vi "read_usalex_photon_hdf5.vi"() -> ()   [LabVIEW 2010]
uses:
  <vilib>/addons/h5labview2/file/H5F.lvlib
  <vilib>/addons/h5labview2/file/H5Fmode.ctl
  <vilib>/addons/h5labview2/group/H5G.lvlib
  <vilib>/addons/h5labview2/dataset/H5Dread.llb/H5Dread.xnode
  <vilib>/addons/h5labview2/base/H5Equery.vi
  <vilib>/addons/h5labview2/base/lib_path.vi
  <vilib>/Analysis/NI_AALBase.lvlib
  <vilib>/Analysis/1siggen.llb/Ramp Pattern by Delta.vi
  <vilib>/addons/h5labview2/base/hid_t.ctl
panel:
  out "measurement_type":string
  out "error out":errorcluster
  out "ALEX Histograms":cluster{"Ramp Pattern":dbl[], u32[]}[](graph)
  out "acceptor_period":u32[](array[numeric])
  out "donor_period":u32[](array[numeric])
  out "alex_offset":u32
  out "alex_period":u32
  out "spectral_ch2":u32[](array[numeric])
  out "spectral_ch1":u32[](array[numeric])
  out "detectors":u32[](array[numeric])
  out "timestamps_unit":dbl
  out "timestamps":i64[](array[numeric])
  in  "Path":path
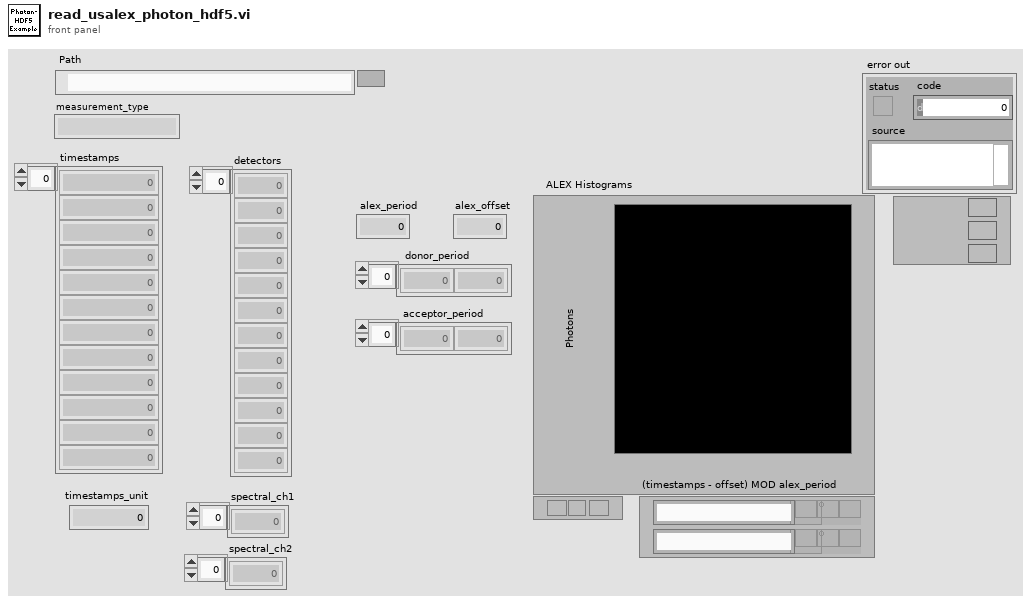
[diagram p1: front panel]
types:
  T1 = typedef "H5F.lvlib/H5Fmode.ctl" = enum16{"read-only", "read-write", "overwrite", "create new", "open or create"}
  T2 = typedef "hid_t.ctl" = i32
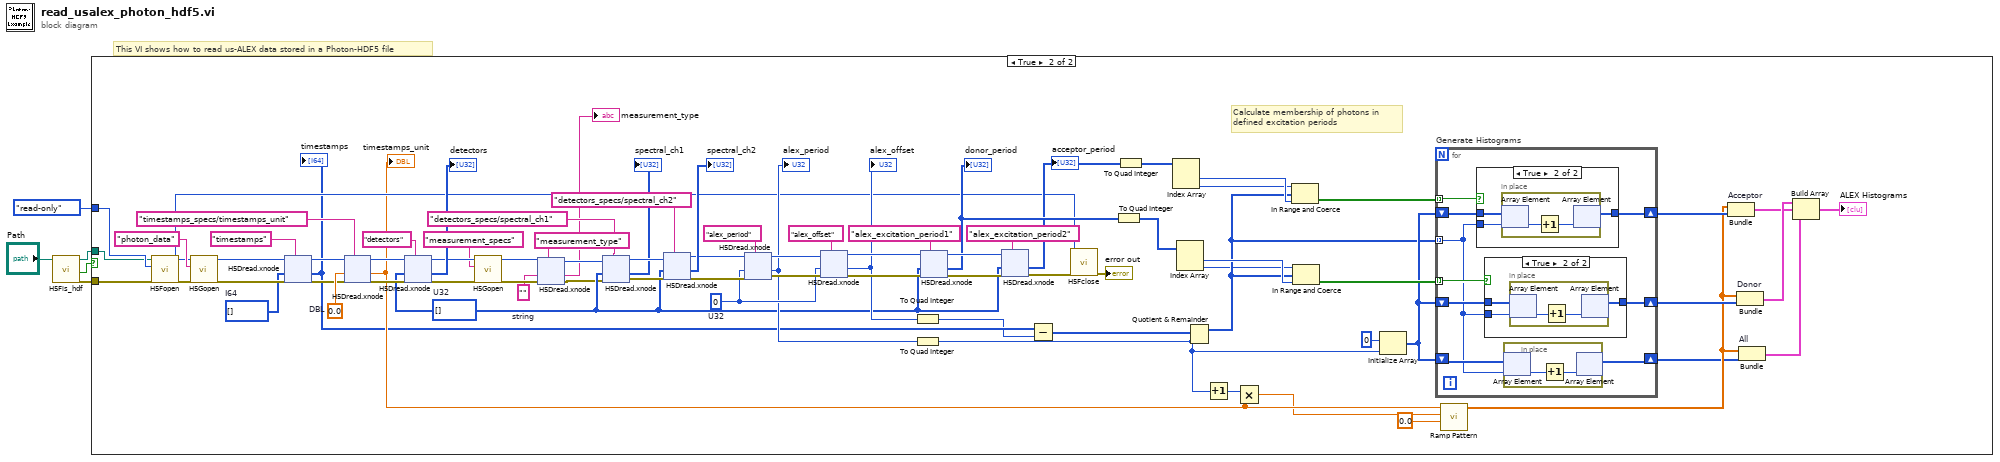
[diagram p0: block diagram]
diagram:
  # "This VI shows how to read us-ALEX data stored in a Photon-HDF5 file"
  n1 = call <vilib>:"H5Fis_hdf.vi"("path in"="Path") -> ("error out"=w1:errorcluster, "valid?"=w2:bool, "path out"=w3:path)  [unwired: 7 in, 1 out]
  n2 = case shown="True" w2 {
    tunnel: H5Fmode."read-only" ("mode (read-only)") -> [_ w86]
    tunnel: w3 -> [_ w85]
    tunnel: w1 -> [_ w84]
    frame False {
    }
    frame True {
      w7 = ""  # string
      w54 = u32 0  # U32
      w37 = u32[] []  # U32
      w77 = 0.0  # DBL
      w78 = i64[] []  # I64
      # "Calculate membership of photons in\ndefined excitation periods"
      n3 = call <vilib>:"H5Fopen.vi"("error in (no error)"=w84, "mode (read-only)"=w86, "path"=w85) -> ("error out"=w83:errorcluster, "ref out"=w32:T2)  [unwired: 7 in]
      n4 = call <vilib>:"H5Gopen.vi"("error in (no error)"=w83, "name"="photon_data", "ref in"=w32) -> ("error out"=w79:errorcluster, "group out"=w81:T2)  [unwired: 7 in]
      n5 = xnode "H5Dread.xnode"("dataset name (this)"="timestamps", "error in (no error)"=w79, "default"=w78, "ref in"=w81) -> ("error out"=w75:errorcluster, "data"=w17:i64[], "ref out"=w76:i32)  [unwired: 2 in, 1 out]
      "timestamps" <- w17
      n6 = xnode "H5Dread.xnode"("dataset name (this)"="timestamps_specs/timestamps_unit" ("object name"), "error in (no error)"=w75, "default"=w77, "ref in"=w76) -> ("error out"=w70:errorcluster, "data"=w29:dbl, "ref out"=w71:i32)  [unwired: 2 in, 1 out]
      "timestamps_unit" <- w29
      n7 = xnode "H5Dread.xnode"("dataset name (this)"="detectors", "error in (no error)"=w70, "default"=w37, "ref in"=w71) -> ("error out"=w67:errorcluster, "data"=→"detectors":u32[], "ref out"=w69:i32)  [unwired: 2 in, 1 out]
      n8 = call <vilib>:"H5Gopen.vi"("error in (no error)"=w67, "name"="measurement_specs" ("object name"), "ref in"=w69) -> ("error out"=w12:errorcluster, "group out"=w10:T2)  [unwired: 7 in]
      n9 = xnode "H5Dread.xnode"("dataset name (this)"="measurement_type" ("object name"), "error in (no error)"=w12, "default"=w7, "ref in"=w10) -> ("error out"=w11:errorcluster, "data"=→"measurement_type":string, "ref out"=w9:i32)  [unwired: 2 in, 1 out]
      n10 = xnode "H5Dread.xnode"("dataset name (this)"="detectors_specs/spectral_ch1", "error in (no error)"=w11, "default"=w37, "ref in"=w9) -> ("error out"=w65:errorcluster, "data"=→"spectral_ch1":u32[], "ref out"=w64:i32)  [unwired: 2 in, 1 out]
      n11 = xnode "H5Dread.xnode"("dataset name (this)"="detectors_specs/spectral_ch2", "error in (no error)"=w65, "default"=w37, "ref in"=w64) -> ("error out"=w59:errorcluster, "data"=→"spectral_ch2":u32[], "ref out"=w60:T2)  [unwired: 2 in, 1 out]
      n12 = xnode "H5Dread.xnode"("dataset name (this)"="alex_period", "error in (no error)"=w59, "default"=w54, "ref in"=w60) -> ("error out"=w56:errorcluster, "data"=w43:u32, "ref out"=w57:i32)  [unwired: 2 in, 1 out]
      "alex_period" <- w43
      n13 = xnode "H5Dread.xnode"("dataset name (this)"="alex_offset", "error in (no error)"=w56, "default"=w54, "ref in"=w57) -> ("error out"=w52:errorcluster, "data"=w47:u32, "ref out"=w53:i32)  [unwired: 2 in, 1 out]
      "alex_offset" <- w47
      n14 = To Quad Integer(1:w47) -> (0:w16:i64)
      n15 = To Quad Integer(1:w43) -> (0:w31:i64)
      n16 = xnode "H5Dread.xnode"("dataset name (this)"="alex_excitation_period1", "error in (no error)"=w52, "default"=w37, "ref in"=w53) -> ("error out"=w49:errorcluster, "data"=w46:u32[], "ref out"=w50:i32)  [unwired: 2 in, 1 out]
      "donor_period" <- w46
      n17 = xnode "H5Dread.xnode"("dataset name (this)"="alex_excitation_period2", "error in (no error)"=w49, "default"=w37, "ref in"=w50) -> ("error out"=w36:errorcluster, "data"=w45:u32[])  [unwired: 2 in, 2 out]
      "acceptor_period" <- w45
      n18 = Subtract(x=w17, y=w16) -> (x-y=w15:i64[])
      n19 = call <vilib>:"H5Fclose.vi"("error in (no error)"=w36, "ref"=w32) -> ("error out"=→"error out":errorcluster)  [unwired: 9 in]
      n20 = To Quad Integer(1:w46) -> (0:w22:i64[])
      n21 = To Quad Integer(1:w45) -> (0:w25:i64[])
      n22 = Index Array(array=w25) -> (element #1=w34:i64, element #2=w33:i64)  [unwired: 2 in]
      n23 = Index Array(array=w22) -> (element #1=w24:i64, element #2=w13:i64)  [unwired: 2 in]
      n24 = Quotient & Remainder(x=w15, y=w31) -> (x-y*floor(x/y)=w14:i64[])  [unwired: 1 out]
      n25 = Increment(x=w31) -> (x+1=w30:i64)
      n26 = Multiply(x=w30, y=w29) -> (x*y=w28:dbl)
      n27 = In Range and Coerce(upper limit=w33, x=w14, lower limit=w34) -> (In Range?=w26:bool[])  [unwired: 1 out]
      n28 = In Range and Coerce(upper limit=w13, x=w14, lower limit=w24) -> (In Range?=w23:bool[])  [unwired: 1 out]
      n29 = Initialize Array(u32 0 ("element"), w31) -> (w19:u32[])
      n30 = for "Generate Histograms" {
        shift-right: [w110] -> w42
        shift-left: w19 -> [w109]
        shift-right: [w107] -> w41
        shift-left: w19 -> [w108]
        tunnel: w14 -> [w102] mode=indexing
        tunnel: w26 -> [w106] mode=indexing
        tunnel: w23 -> [w105] mode=indexing
        shift-right: [w103] -> w18
        shift-left: w19 -> [w104]
        n31 = case shown="True" w106 {
          tunnel: [w119 w120] -> w110
          tunnel: w109 -> [w119 w122]
          tunnel: w102 -> [_ w121]
          frame False {
          }
          frame True {
            n32 = in-place {
              n33 = in-place-array #1(w122, w121) -> (w124:u32)
              n34 = Increment(x=w124) -> (x+1=w123:u32)
              n35 = in-place-array #1(w123) -> (w120:u32[])  [unwired: 1 out]
            }
          }
        }
        n36 = case shown="True" w105 {
          tunnel: [w113 w114] -> w107
          tunnel: w108 -> [w113 w116]
          tunnel: w102 -> [_ w115]
          frame False {
          }
          frame True {
            n37 = in-place {
              n38 = in-place-array #2(w116, w115) -> (w118:u32)
              n39 = Increment(x=w118) -> (x+1=w117:u32)
              n40 = in-place-array #2(w117) -> (w114:u32[])  [unwired: 1 out]
            }
          }
        }
        n41 = in-place {
          n42 = in-place-array #3(w104, w102) -> (w112:u32)
          n43 = Increment(x=w112) -> (x+1=w111:u32)
          n44 = in-place-array #3(w111) -> (w103:u32[])  [unwired: 1 out]
        }
      }
      n45 = call-poly <vilib>:"Ramp Pattern.vi"("start"=0.0, "end"=w28, "delta"=w29) -> ("Ramp Pattern"=w21:dbl[])  [unwired: 6 in, 2 out]
      n46 = Bundle "Acceptor"("Ramp Pattern"=w21, w42) -> (w39:cluster{"Ramp Pattern":dbl[], u32[]})  [unwired: 1 in]
      n47 = Bundle "Donor"("Ramp Pattern"=w21, w41) -> (w40:cluster{"Ramp Pattern":dbl[], u32[]})  [unwired: 1 in]
      n48 = Bundle "All"("Ramp Pattern"=w21, w18) -> (w20:cluster{"Ramp Pattern":dbl[], u32[]})  [unwired: 1 in]
      n49 = Build Array(w40, w39, w20) -> (→"ALEX Histograms":cluster{"Ramp Pattern":dbl[], u32[]}[])
    }
  }
